vi "RSZVB Trace Get Channel Name.vi"(8 "error in (no error)":errorcluster {"code" format="%.0x"}, 10 "Trace Name (Ch2Trc2)":string="Ch2Trc2", 11 "VISA session":refnum<visa-resource-name>) -> (0 "error out":errorcluster {"code" format="%.0x"}, 2 "Channel Name":string, 3 "dup VISA session":refnum<visa-resource-name>)   [LabVIEW 2011]
doc: "This VI returns the channel name for an existing trace named '<Trc_name>'. \n\nRemote-control command(s):\nCONFigure:TRACe:CHANnel:NAME? '<Trc_name>'"
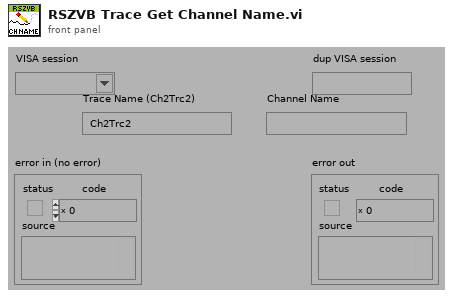
[diagram p1: front panel]
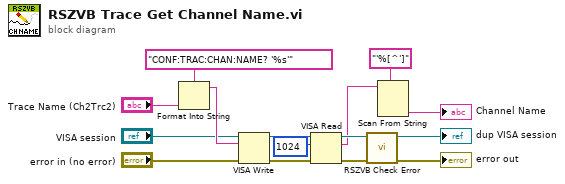
[diagram p0: block diagram]
diagram:
  n1 = Format Into String(format string="CONF:TRAC:CHAN:NAME? '%s'", "Trace Name (Ch2Trc2)") -> (resulting string=w9:string)  [unwired: 2 in, 1 out]
  n2 = VISA Write(VISA resource name="VISA session", write buffer=w9, error in (no error)="error in (no error)") -> (VISA resource name out=w11:refnum<visa-resource-name>, error out=w12:errorcluster)  [unwired: 1 out]
  n3 = VISA Read(VISA resource name=w11, byte count=u32 1024 ("byte count (0)"), error in (no error)=w12) -> (VISA resource name out=w14:refnum<visa-resource-name>, read buffer=w7:string, error out=w13:errorcluster)  [unwired: 1 out]
  n4 = call "RSZVB Check Error.vi"("error in (no error)"=w13, "VISA session"=w14) -> ("error out"=→"error out":errorcluster, "dup VISA session"=→"dup VISA session":refnum<visa-resource-name>)  [unwired: 8 in]
  n5 = Scan From String(format string="'%[^']", input string=w7) -> (output 1=→"Channel Name":string)  [unwired: 3 in, 3 out]
